vi "_ReadAttributes.vi"(0 "device name":string, 1 "attribute names":string[](array[string])) -> (2 "attribute values":T3(array[cluster]), 3 "error code":i32, 4 "error stack":string[](array[string]))   [LabVIEW 2017, in "tango.lvlib"]
uses:
  tango.lvlib
  Common VIs/Typedefs/_AttributeQuality_t.ctl
  Common VIs/Typedefs/_AttributeDataType_t.ctl
  tango_binding.dll
panel:
  # "This Vi is deprecated and only maintained for backward compatibility. Please use  _TangoReadAttributes instead."
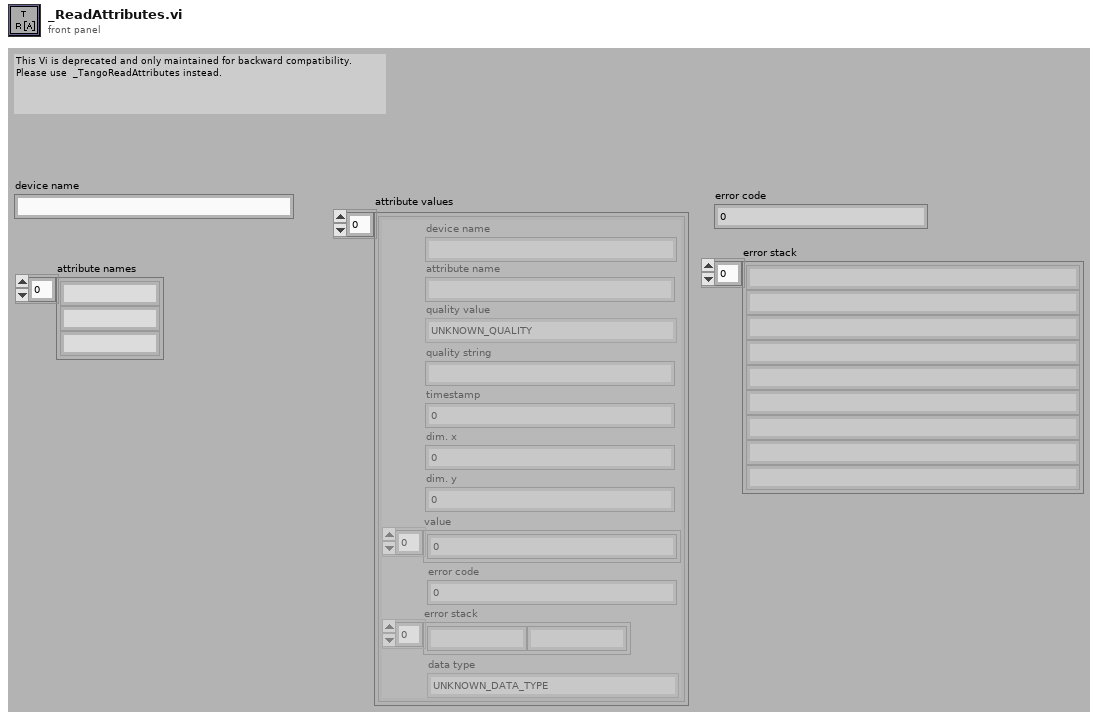
[diagram p1: front panel]
types:
  T1 = typedef "tango.lvlib/_AttributeQuality_t.ctl" = enum16{"VALID", "INVALID", "ALARM", "CHANGING", "UNKNOWN_QUALITY"}
  T2 = typedef "tango.lvlib/_AttributeDataType_t.ctl" = enum16{"STATE_SCA", "STATE_SPE", "STATE_IMG", "STRING_SCA", "STRING_SPE", "STRING_IMG", "BOOL_SCA", "BOOL_SPE", "BOOL_IMG", "UCHAR_SCA", "UCHAR_SPE", "UCHAR_IMG", "SHORT_SCA", "SHORT_SPE", "SHORT_IMG", "USHORT_SCA", "USHORT_SPE", "USHORT_IMG", "LONG_SCA", "LONG_SPE", "LONG_IMG", "ULONG_SCA", "ULONG_SPE", "ULONG_IMG", "LONG64_SCA", "LONG64_SPE", "LONG64_IMG", "ULONG64_SCA", "ULONG64_SPE", "ULONG64_IMG", "FLOAT_SCA", "FLOAT_SPE", "FLOAT_IMG", "DOUBLE_SCA", "DOUBLE_SPE", "DOUBLE_IMG", "ENUM_SCA", "UNKNOWN_DATA_TYPE"}
  T3 = cluster{"device name":string, "attribute name":string, "quality value":T1, "quality string":string, "timestamp":dbl, "dim. x":i32, "dim. y":i32, "value":u8[], "error code":i32, "error stack":string[], "data type":T2}[]
  T4 = typedef "tango.lvlib/_AttributeValue_t.ctl" = cluster{"device name":string, "attribute name":string, "quality value":T1, "quality string":string, "timestamp":dbl, "dim. x":i32, "dim. y":i32, "value":u8[], "error code":i32, "error stack":string[], "data type":T2}
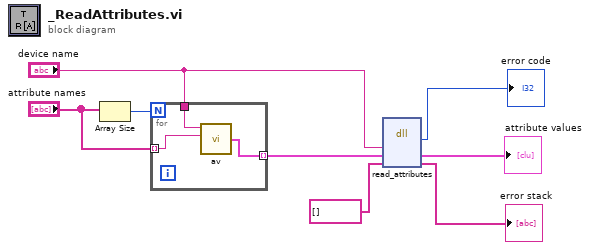
[diagram p0: block diagram]
diagram:
  n1 = Array Size(array="attribute names") -> (size(s)=w3:i32)
  n2 = for {
    N: w3 -> [_]
    tunnel: "device name" -> [w10]
    tunnel: "attribute names" -> [w9] mode=indexing
    tunnel: [w11] -> w2 mode=indexing
    n3 = call "av.vi"("attribute name"=w9, "device name"=w10) -> ("attribute value"=w11:T4)  [unwired: 4 in]
  }
  n4 = dll-call lib="tango_binding.*" fn="read_attributes"("dev_name"="device name", "attr_values_inout"=w2, "error_stack"=string[] [] ("error stack")) -> ("return type"=→"error code":i32, "attr_values_inout"=→"attribute values":T4[], "error_stack"=→"error stack":string[])  [unwired: 4 in, 2 out]
